vi "SeCrTs-AI_Config_Divide.vi"(11 "AI config":T1(array[cluster])) -> (1 "AI C":T1(array[cluster]), 3 "AI V":T1(array[cluster]))   [LabVIEW 2022 SP3]
panel:
  in  "V_DAQ Card 2":string="PXI1Slot7"
  in  "V_DAQ Card":string="Mod4"
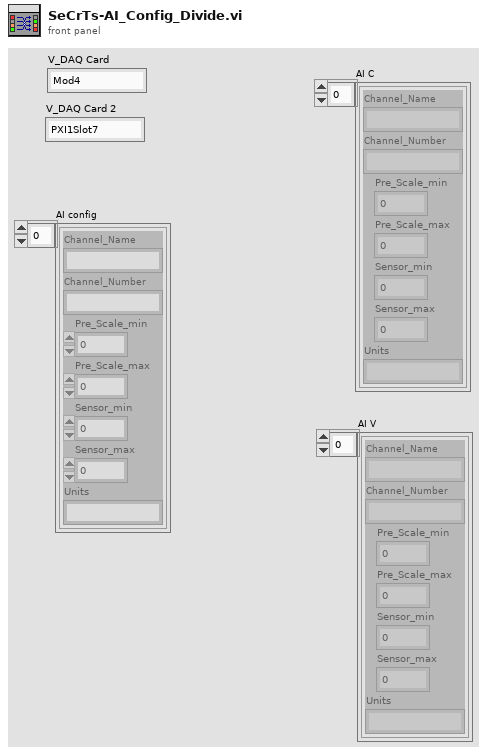
[diagram p1: front panel]
types:
  T1 = cluster{"Channel_Name":string, "Channel_Number":string, "Pre_Scale_min":dbl, "Pre_Scale_max":dbl, "Sensor_min":dbl, "Sensor_max":dbl, "Units":string}[]
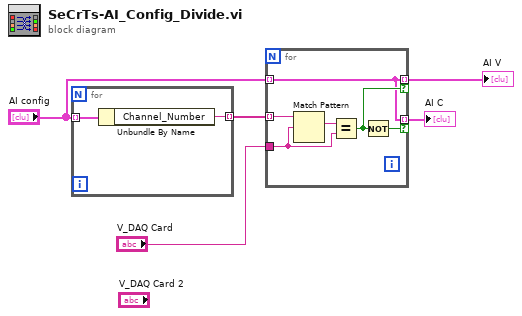
[diagram p0: block diagram]
diagram:
  n1 = for {
    tunnel: "AI config" -> [w7] mode=indexing
    tunnel: [w6] -> w4 mode=indexing
    n2 = Unbundle By Name(w7) -> ("Channel_Number"=w6:string)
  }
  n3 = for {
    tunnel: "V_DAQ Card" -> [w12]
    tunnel: [w8] -> w2 mode=indexing if=w11
    tunnel: [w8] -> w3 mode=indexing if=w10
    tunnel: w4 -> [w9] mode=indexing
    tunnel: "AI config" -> [w8] mode=indexing
    n4 = Match Pattern(string=w9, regular expression=w12) -> (match substring=w13:string)  [unwired: 1 in, 3 out]
    n5 = Equal?(x=w13, y=w12) -> (x = y?=w11:bool)
    n6 = Not(x=w11) -> (.not. x?=w10:bool)
  }
  "AI C" <- w3
  "AI V" <- w2
